vi "Write_Calibrations_to_File.vi"   [LabVIEW 2018]
uses:
  Global_Variables/Dashboard_Globals.vi
types:
  T1 = enum16{"open", "replace", "create", "open or create", "replace or create", "replace or create with confirmation"}
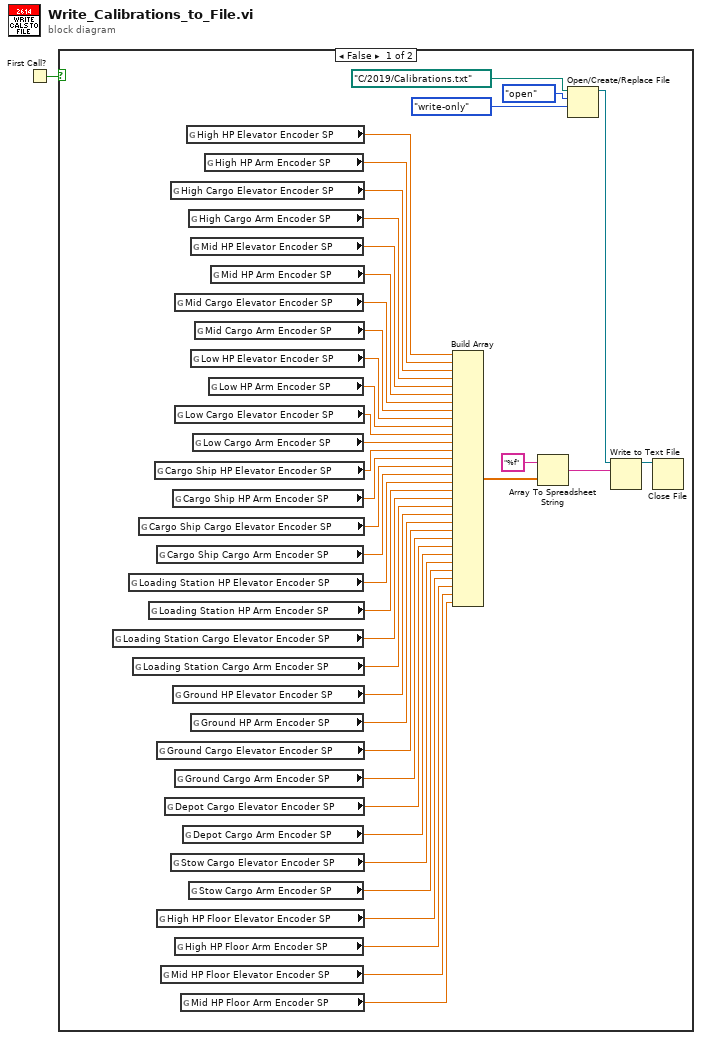
[diagram p0: block diagram]
diagram:
  n1 = First Call?() -> (First Call?: T/F=w1:bool)
  n2 = case shown="False" w1 {
    frame False {
      n3 = global read "Dashboard_Globals.vi" "Loading Station Cargo Elevator Encoder SP"() -> (w15:dbl)
      n4 = global read "Dashboard_Globals.vi" "Loading Station HP Elevator Encoder SP"() -> (w17:dbl)
      n5 = global read "Dashboard_Globals.vi" "Loading Station Cargo Arm Encoder SP"() -> (w14:dbl)
      n6 = global read "Dashboard_Globals.vi" "Cargo Ship Cargo Elevator Encoder SP"() -> (w19:dbl)
      n7 = global read "Dashboard_Globals.vi" "Loading Station HP Arm Encoder SP"() -> (w16:dbl)
      n8 = global read "Dashboard_Globals.vi" "Cargo Ship HP Elevator Encoder SP"() -> (w21:dbl)
      n9 = global read "Dashboard_Globals.vi" "Cargo Ship Cargo Arm Encoder SP"() -> (w18:dbl)
      n10 = global read "Dashboard_Globals.vi" "Ground Cargo Elevator Encoder SP"() -> (w11:dbl)
      n11 = global read "Dashboard_Globals.vi" "High HP Floor Elevator Encoder SP"() -> (w5:dbl)
      n12 = global read "Dashboard_Globals.vi" "Mid HP Floor Elevator Encoder SP"() -> (w3:dbl)
      n13 = global read "Dashboard_Globals.vi" "Depot Cargo Elevator Encoder SP"() -> (w9:dbl)
      n14 = global read "Dashboard_Globals.vi" "High Cargo Elevator Encoder SP"() -> (w31:dbl)
      n15 = global read "Dashboard_Globals.vi" "Stow Cargo Elevator Encoder SP"() -> (w7:dbl)
      n16 = global read "Dashboard_Globals.vi" "Cargo Ship HP Arm Encoder SP"() -> (w20:dbl)
      n17 = global read "Dashboard_Globals.vi" "Ground HP Elevator Encoder SP"() -> (w13:dbl)
      n18 = global read "Dashboard_Globals.vi" "Mid Cargo Elevator Encoder SP"() -> (w27:dbl)
      n19 = global read "Dashboard_Globals.vi" "Low Cargo Elevator Encoder SP"() -> (w23:dbl)
      n20 = global read "Dashboard_Globals.vi" "Ground Cargo Arm Encoder SP"() -> (w10:dbl)
      n21 = global read "Dashboard_Globals.vi" "High HP Floor Arm Encoder SP"() -> (w4:dbl)
      n22 = global read "Dashboard_Globals.vi" "Mid HP Floor Arm Encoder SP"() -> (w2:dbl)
      n23 = global read "Dashboard_Globals.vi" "Depot Cargo Arm Encoder SP"() -> (w8:dbl)
      n24 = global read "Dashboard_Globals.vi" "High HP Elevator Encoder SP"() -> (w33:dbl)
      n25 = global read "Dashboard_Globals.vi" "High Cargo Arm Encoder SP"() -> (w30:dbl)
      n26 = global read "Dashboard_Globals.vi" "Stow Cargo Arm Encoder SP"() -> (w6:dbl)
      n27 = global read "Dashboard_Globals.vi" "Mid HP Elevator Encoder SP"() -> (w29:dbl)
      n28 = global read "Dashboard_Globals.vi" "Low HP Elevator Encoder SP"() -> (w25:dbl)
      n29 = global read "Dashboard_Globals.vi" "Ground HP Arm Encoder SP"() -> (w12:dbl)
      n30 = global read "Dashboard_Globals.vi" "Low Cargo Arm Encoder SP"() -> (w22:dbl)
      n31 = global read "Dashboard_Globals.vi" "Mid Cargo Arm Encoder SP"() -> (w26:dbl)
      n32 = global read "Dashboard_Globals.vi" "High HP Arm Encoder SP"() -> (w32:dbl)
      n33 = global read "Dashboard_Globals.vi" "Low HP Arm Encoder SP"() -> (w24:dbl)
      n34 = global read "Dashboard_Globals.vi" "Mid HP Arm Encoder SP"() -> (w28:dbl)
      n35 = Build Array(w33, w32, w31, w30, w29, w28, w27, w26, w25, w24, w23, w22, w21, w20, w19, w18, w17, w16, w15, w14, w13, w12, w11, w10, w9, w8, w7, w6, w5, w4, w3, w2) -> (w34:dbl[])
      n36 = Array To Spreadsheet String(array=w34, 3:"%f" ("format string")) -> (spreadsheet string=w35:string)  [unwired: 1 in]
      n37 = Open/Create/Replace File(file path (use dialog)=path "C:/2019/Calibrations.txt" ("file (use dialog)"), operation (0:open)=T1."open", access (0:read/write)=enum16{"read/write", "read-only", "write-only"}."write-only") -> (refnum out=w40:refnum<file>)  [unwired: 3 in, 2 out]
      n38 = Write to Text File(file (use dialog)=w40, text=w35) -> (refnum out=w41:refnum<file>)  [unwired: 2 in, 2 out]
      n39 = Close File(refnum=w41) -> ()  [unwired: 1 in, 2 out]
    }
    frame True {
    }
  }
